vi "OGB Replace Keywords in File.vi"(8 "error in (no error)":errorcluster, 9 "Values":string[](array[string]), 10 "Keywords":string[](array[string]), 11 "file path":path) -> (0 "error out":errorcluster, 3 "dup file path":path)   [LabVIEW 2011]
uses:
  <userlib>/_OpenG.lib/file/file.llb/Valid Path__ogtk.vi
  <userlib>/_OpenG.lib/file/file.llb/File Exists - Scalar__ogtk.vi
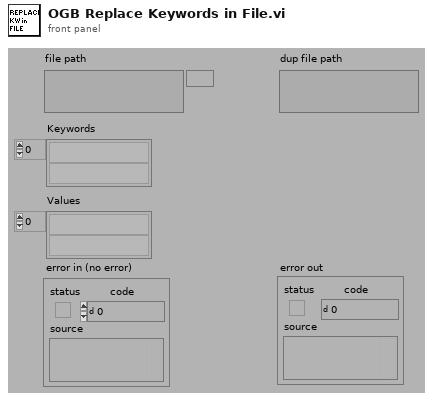
[diagram p1: front panel]
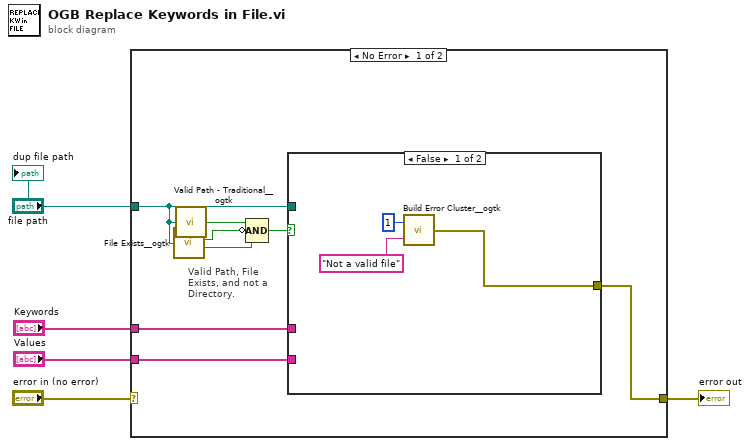
[diagram p0: block diagram]
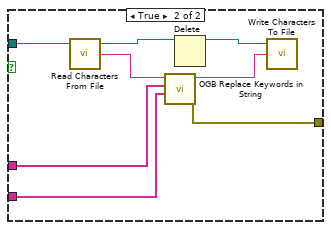
[diagram p2: hidden frame]
diagram:
  n1 = case shown="No Error" "error in (no error)" {
    selector: "error in (no error)" -> [_ w25]
    tunnel: "file path" -> [w13 _]
    tunnel: [w8 w25] -> w5
    tunnel: "Keywords" -> [w7 _]
    tunnel: "Values" -> [w6 _]
    frame No Error {
      # "Valid Path, File Exists, and not a Directory."
      n2 = call-poly <userlib>:"File Exists__ogtk.vi"("file path"=w13) -> ("is directory"=w10:bool, "exists"=w11:bool)  [unwired: 6 in]
      n3 = call-poly <userlib>:"Valid Path - Traditional__ogtk.vi"("path"=w13) -> ("valid"=w12:bool)
      n4 = Compound Arithmetic op=AND(w12, invert w10, w11) -> (w9:bool)
      n5 = case shown="False" w9 {
        tunnel: w13 -> [_ w22]
        tunnel: [w14 w21] -> w8
        tunnel: w7 -> [_ w20]
        tunnel: w6 -> [_ w19]
        frame False {
          n6 = call <userlib>:"Build Error Cluster__ogtk.vi"("String to Prepend to source (\"\")"="Not a valid file" ("String to Prepend to source (\"\")"), "code"=1) -> ("error out"=w14:errorcluster)
        }
        frame True {
          n7 = call <vilib>:"Read Characters From File.vi"("file path (dialog if empty)"=w22) -> ("new file path (NotAPath if cancelled)"=w18:path, "character string"=w24:string)  [unwired: 5 in, 2 out]
          n8 = call "OGB Replace Keywords in String.vi"("Value"=w19, "Keyword"=w20, "String in"=w24) -> ("error out"=w21:errorcluster, "String out"=w23:string)  [unwired: 7 in]
          n9 = Delete(path (use dialog)=w18) -> (deleted path=w17:path)  [unwired: 4 in, 2 out]
          n10 = call <vilib>:"Write Characters To File.vi"("character string"=w23, "file path (dialog if empty)"=w17) -> ()  [unwired: 3 in, 1 out]
        }
      }
    }
    frame Error {
    }
  }
  "error out" <- w5
  "dup file path" <- "file path"
